vi "Bury All Target.vi"() -> ()   [LabVIEW 2017, in "Tests.lvlib" / "Bookmark Manager.lvlib"]
uses:
  Bookmark Manager.lvlib
panel:
  in  "Input 3":bool[](array[boolean])=[FALSE, FALSE, FALSE, TRUE, FALSE, FALSE]
  out "Any? 3":bool
  in  "Input 2":bool[](array[boolean])=[FALSE, FALSE, FALSE, TRUE, FALSE, FALSE]
  out "Any? 2":bool
  in  "Input 1":bool[](array[boolean])=[FALSE, FALSE, FALSE, TRUE, FALSE, FALSE]
  out "Any? 1":bool
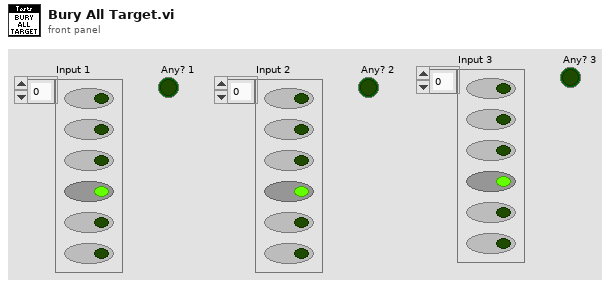
[diagram p1: front panel]
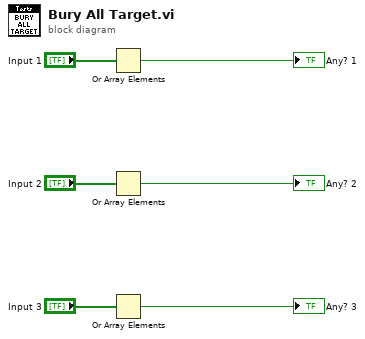
[diagram p0: block diagram]
diagram:
  n1 = Or Array Elements(Boolean array="Input 1") -> (logical OR=→"Any? 1":bool)
  n2 = Or Array Elements(Boolean array="Input 2") -> (logical OR=→"Any? 2":bool)
  n3 = Or Array Elements(Boolean array="Input 3") -> (logical OR=→"Any? 3":bool)
